vi "FileSave.vi"(8 "error in":errorcluster caption="에러 입력(에러 없음)", 10 "Array Size":i32, 11 "File Path":string) -> (0 "error out":errorcluster caption="에러 출력", 3 "Random Array":dbl[](array[numeric]))   [LabVIEW 2014]
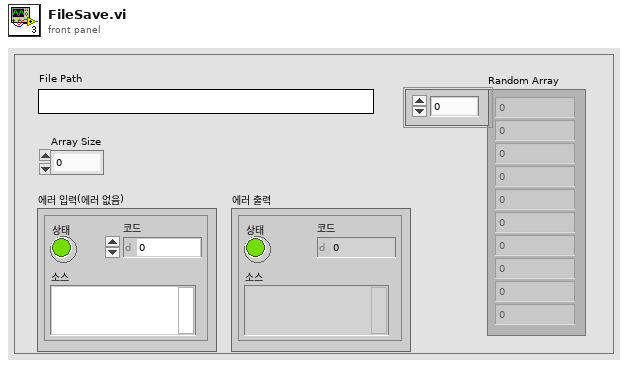
[diagram p1: front panel]
types:
  T1 = enum16{"open", "replace", "create", "open or create", "replace or create", "replace or create with confirmation"}
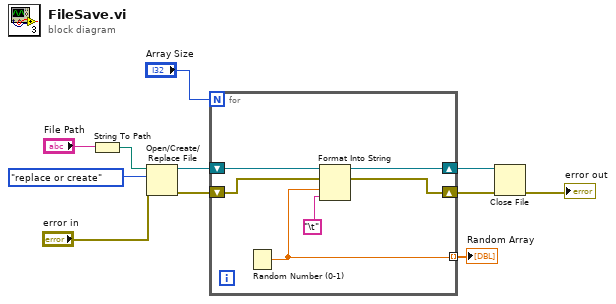
[diagram p0: block diagram]
diagram:
  n1 = String To Path(string="File Path") -> (path=w10:path)
  n2 = Open/Create/Replace File(file path (use dialog)=w10, error in="error in", operation (0:open)=T1."replace or create" ("동작(0:open)")) -> (refnum out=w8:refnum<file>, error out=w7:errorcluster)  [unwired: 3 in, 1 out]
  n3 = for {
    N: "Array Size" -> [_]
    shift-right: [w16] -> w4
    shift-left: w8 -> [w17]
    shift-right: [w14] -> w3
    shift-left: w7 -> [w15]
    tunnel: [w12] -> w5 mode=indexing
    n4 = Random Number (0-1)() -> (number: 0 to 1=w12:dbl)
    n5 = Format Into String(initial string=w17, error in=w15, w12, "\t") -> (resulting string=w16:refnum<file>, error out=w14:errorcluster)  [unwired: 1 in]
  }
  "Random Array" <- w5
  n6 = Close File(refnum=w4, error in=w3) -> (error out=→"error out":errorcluster)  [unwired: 1 out]
